vi "CHS-simulate-robot-on-field.vi"() -> ()   [LabVIEW 2019]
uses:
  <vilib>/Rock Robotics/WPI/Camera/WPI_CameraImageSize.ctl
  <vilib>/Rock Robotics/WPI/ThirdParty/JAS_Junk/TrajLib/TypeDef/FieldDisp_ElementPicture.ctl
  <vilib>/Rock Robotics/WPI/ThirdParty/JAS_Junk/TrajLib/VI/FieldDisp_Element_Rotate.vi
  <vilib>/Rock Robotics/WPI/ThirdParty/JAS_Junk/TrajLib/Conv_Meters_Inches.vi
  <vilib>/Rock Robotics/WPI/ThirdParty/JAS_Junk/TrajLib/Conv_Radians_Deg.vi
  Simulation/CHS_SIM_SIM_Globals.vi
  <vilib>/picture/pixmap.llb/Flatten Pixmap.vi
  <vilib>/picture/pictutil.llb/Create Mask.vi
  <vilib>/picture/picture.llb/Draw Flattened Pixmap.vi
  SubVI/CHS_Robot Global Data.vi
  <vilib>/Rock Robotics/WPI/ThirdParty/JAS_Junk/TrajLib/Trajectory_Library.lvlib
panel:
  out "ROBOT 2":T1
  in  "Finish":bool
  in  "Enable Vision":bool
  in  "Image Size":T2=enum."320x240"
  out "Field Picture":picture
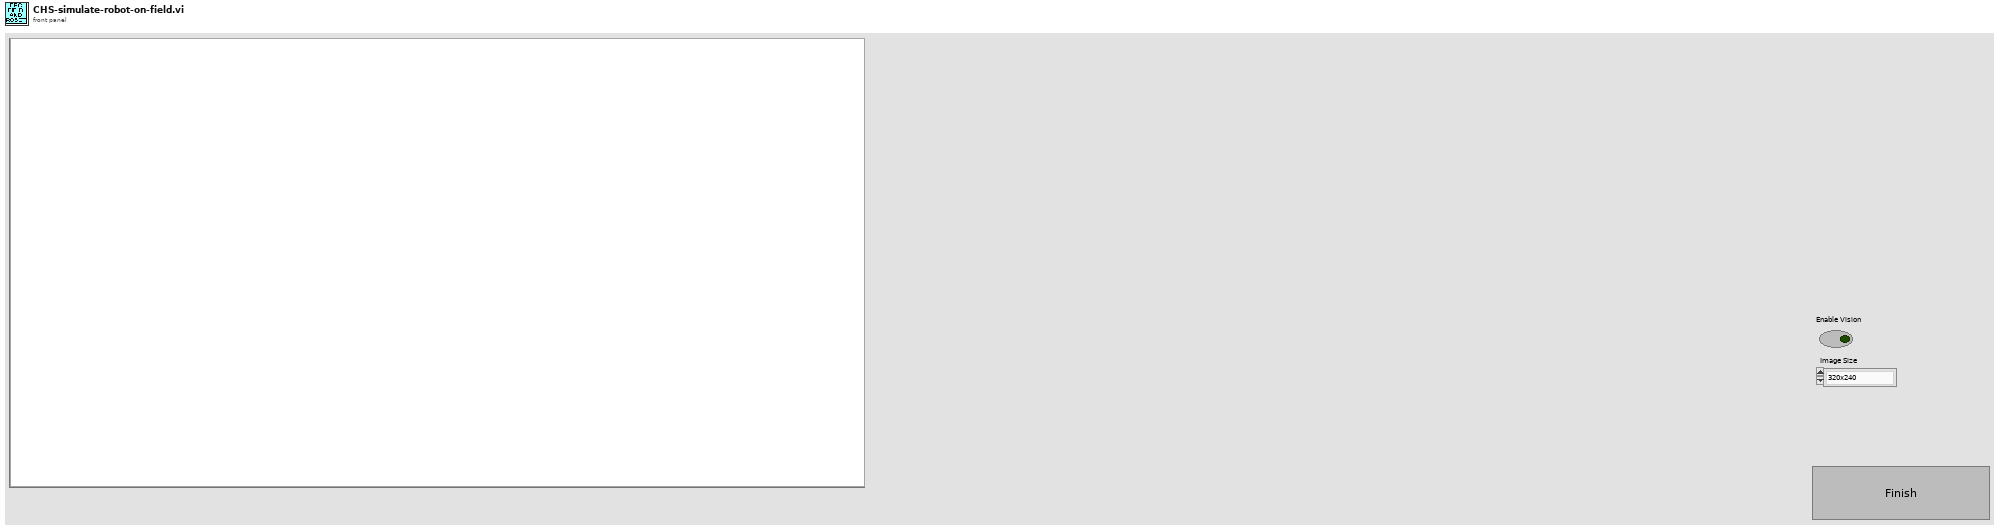
[diagram p1: front panel]
types:
  T1 = typedef "Trajectory_Library.lvlib/FieldDisp_ElementPicture.ctl" = picture
  T2 = typedef "WPI_CameraImageSize.ctl" = enum16{"640x480", "320x240", "160x120", "Custom"}
  T3 = typedef "WPI_DriverStationMatch Info.ctl" = cluster{"Autonomous Elapsed Seconds":dbl, "TeleOp Elapsed Seconds":dbl, "Disabled Elapsed Seconds":dbl, "Visited Autonomous":bool, "Visited TeleOp":bool, "Visited Disabled":bool, "Autonomous Settings":cluster{"Autonomous Style":enum16{"Iterative", "Independent"}, "VI Refnum":refnum<vi>}}
  T4 = typedef "WPI_DriverStationDerivedRobotMode.ctl" = enum16{"Init", "Execute", "Stop"}
  T5 = typedef "WPI_DriverStationRobotMode2.ctl" = enum16{"Autonomous Disabled", "Autonomous Enabled", "Teleop Disabled", "Teleop Enabled", "Disconnected", "Finish", "Test Disabled", "Test Enabled", "Emergency Stopped"}
  T6 = typedef "Trajectory_Library.lvlib/FieldDisp_FieldElement.ctl" = cluster{"ONE-8-bit pixmap":u8[][], "Two-Array":cdb[][], "Three-Numeric":i32, "Four-Numeric":i32, "Five-Numeric":cdb, "Six-colors":u32[], "Seven-new element/subarray":u32, "Left Pixel":dbl, "Top Pixel":dbl, "Width Pix/Ft":dbl, "Height Pix/Ft":dbl, "Element Picture Ref":refnum<vi>}
  T7 = typedef "Trajectory_Library.lvlib/SWERVE_DRIVE_ODOMETRY.ctl" = cluster{"POSE":T8, "GyroOffset":T10, "PreviousAngle":T10, "PrevModulePositions":T11[], "NumModules":i32}
  T8 = typedef "Trajectory_Library.lvlib/POSE2D.ctl" = cluster{"TRANSLATION":T9, "ROTATION":T10}
  T9 = typedef "Trajectory_Library.lvlib/TRANSLATION2D.ctl" = cluster{"X":dbl, "Y":dbl}
  T10 = typedef "Trajectory_Library.lvlib/ROTATION2D.ctl" = cluster{"VALUE":dbl, "COS":dbl, "SIN":dbl}
  T11 = typedef "Trajectory_Library.lvlib/SWERVE_DRIVE_MODULE_POSITION.ctl" = cluster{"Distance":dbl, "Angle":T10, "P":bool}
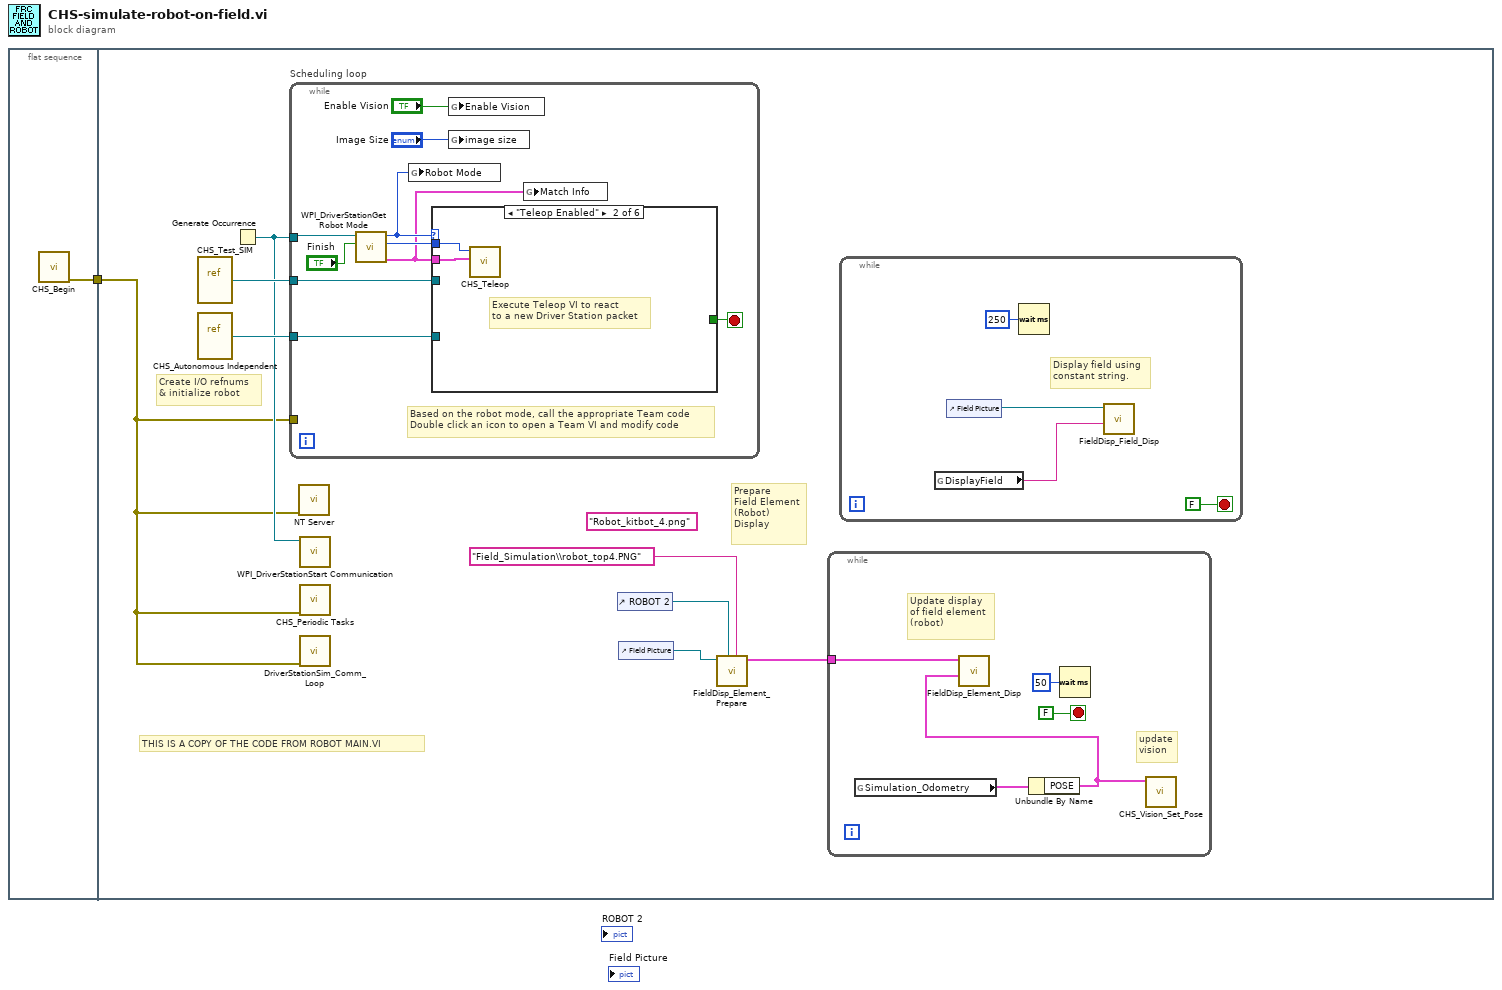
[diagram p0: block diagram]
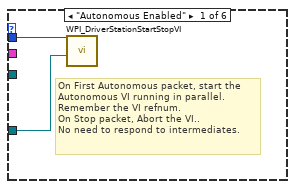
[diagram p2: hidden frame]
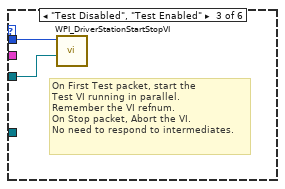
[diagram p3: hidden frame]
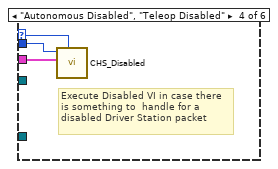
[diagram p4: hidden frame]
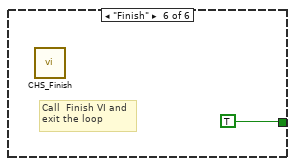
[diagram p6: hidden frame]
diagram:
  n1 = flat-sequence {
    tunnel: [w2] -> w1
    tunnel: w1 -> [w3]
    frame #0 {
      n2 = call "CHS_Begin.vi"() -> ("error out"=w2:errorcluster)  [unwired: 11 in]
    }
    frame #1 {
      (unwired) "Robot_kitbot_4.png" ("Picture FIle Name")
      # "Prepare\nField Element\n(Robot)\nDisplay"
      # "THIS IS A COPY OF THE CODE FROM ROBOT MAIN.VI"
      # "Create I/O refnums\n& initialize robot"
      n3 = vi-ref "CHS_Test_SIM.vi"() -> (w9:refnum<vi>)
      n4 = vi-ref "CHS_Autonomous Independent.vi"() -> (w10:refnum<vi>)
      n5 = Generate Occurrence() -> (w8:refnum<k4>)
      n6 = while "Scheduling loop" {
        tunnel: w8 -> [w28]
        tunnel: w3 -> [_]
        tunnel: w10 -> [w24]
        tunnel: w9 -> [w22]
        stop <- w26 stop-if-true
        # "Based on the robot mode, call the appropriate Team code\nDouble click an icon to open a Team VI and modify code"
        n7 = call <vilib>:"WPI_DriverStationGet Robot Mode.vi"("Finish"="Finish", "DS Occurrence"=w28) -> ("Match Info out"=w20:T3, "Call Context"=w29:T4, "Robot Mode"=w21:T5)  [unwired: 7 out]
        n8 = global write "CHS_Robot Global Data.vi" "Robot Mode"(w21) -> ()
        n9 = case shown="\"Teleop Enabled\"" w21 {
          selector: w21 -> [_ _ _ w36 _ _]
          tunnel: w29 -> [w31 w33 w35 w38 _ _]
          tunnel: w20 -> [_ w32 _ w37 _ _]
          tunnel: [_ _ _ _ _ TRUE] -> w26
          tunnel: w24 -> [w30 _ _ _ _ _]
          tunnel: w22 -> [_ _ w34 _ _ _]
          frame "Autonomous Enabled" {
            # "On First Autonomous packet, start the\nAutonomous VI running in parallel.\nRemember the VI refnum.\nOn Stop packet, Abort the VI..\nNo need to respond to intermediates."
            n10 = call <vilib>:"WPI_DriverStationStartStopVI.vi"("VI in"=w30, "Call Context"=w31) -> ()  [unwired: 10 in]
          }
          frame "Teleop Enabled" {
            # "Execute Teleop VI to react\nto a new Driver Station packet"
            n11 = call "CHS_Teleop.vi"("Match Info"=w32, "Call Context"=w33) -> ()  [unwired: 1 in, 9 out]
          }
          frame "Test Disabled", "Test Enabled" {
            # "On First Test packet, start the\nTest VI running in parallel.\nRemember the VI refnum.\nOn Stop packet, Abort the VI.\nNo need to respond to intermediates."
            n12 = call <vilib>:"WPI_DriverStationStartStopVI.vi"("VI in"=w34, "Call Context"=w35) -> ()  [unwired: 10 in]
          }
          frame "Autonomous Disabled", "Teleop Disabled" {
            # "Execute Disabled VI in case there\nis something to  handle for a\ndisabled Driver Station packet"
            n13 = call "CHS_Disabled.vi"("Robot Mode"=w36, "Match Info"=w37, "Call Context"=w38) -> ()  [unwired: 1 in, 8 out]
          }
          frame "Disconnected", Default {
            # "Driver Station packet didn't arrive.\nPossibly useful for diagnostics"
          }
          frame "Finish" {
            # "Call  Finish VI and\nexit the loop"
            n14 = call "CHS_Finish.vi"() -> ()  [unwired: 1 in, 7 out]
          }
        }
        n15 = global write "CHS_Robot Global Data.vi" "Enable Vision"("Enable Vision") -> ()
        n16 = global write "CHS_Robot Global Data.vi" "image size"("Image Size") -> ()
        n17 = global write "CHS_Robot Global Data.vi" "Match Info"(w20) -> ()
      }
      n18 = call <vilib>:"NT Server.vi"("error in (no error)"=w3) -> ()  [unwired: 10 in, 1 out]
      n19 = call <vilib>:"WPI_DriverStationStart Communication.vi"("occurrence"=w8) -> ()  [unwired: 2 in, 9 out]
      n20 = call "CHS_Periodic Tasks.vi"("error in"=w3) -> ()  [unwired: 11 in]
      n21 = call <vilib>:"DriverStationSim_Comm_Loop.vi"("error in (no error)"=w3) -> ()  [unwired: 11 in]
      n22 = control-ref of="ROBOT 2"() -> (w6:refnum<vi>)
      n23 = control-ref of="Field Picture"() -> (w7:refnum<vi>)
      n24 = call <vilib>:"FieldDisp_Element_Prepare.vi"("Element File Name"="Field_Simulation\\robot_top4.PNG" ("name or relative path"), "Element Picture Ref"=w6, "Field Picture Ref"=w7) -> ("Field Element Info"=w5:T6)  [unwired: 7 in, 1 out]
      n25 = while {
        tunnel: w5 -> [w17]
        stop <- FALSE stop-if-true
        # "update\nvision"
        # "Update display\nof field element\n(robot)"
        n26 = global read "CHS_SIM_SIM_Globals.vi" "Simulation_Odometry"() -> (w16:T7)
        n27 = Unbundle By Name(w16) -> ("POSE"=w15:T8)
        n28 = call <vilib>:"FieldDisp_Element_Disp.vi"("Element Pose"=w15, "Element Info"=w17) -> ()  [unwired: 10 in]
        n29 = Wait (ms)(milliseconds to wait=u32 50) -> ()  [unwired: 1 out]
        n30 = call "CHS_Vision_Set_Pose.vi"("Vison Pose"=w15) -> ()  [unwired: 11 in]
      }
      n31 = while {
        stop <- FALSE stop-if-true
        # "Display field using\nconstant string."
        n32 = global read "CHS_Robot Global Data.vi" "DisplayField"() -> (w11:string)
        n33 = control-ref of="Field Picture"() -> (w14:refnum<vi>)
        n34 = Wait (ms)(milliseconds to wait=u32 250) -> ()  [unwired: 1 out]
        n35 = call <vilib>:"FieldDisp_Field_Disp.vi"("Field Selector"=w11, "Picture in"=w14) -> ()  [unwired: 9 in, 1 out]
      }
    }
  }
